vi "validate configuration.vi"(8 "error in":errorcluster, 11 "Tag Bus Web Interface configuration in":refnum<class "Tag Bus Web Interface configuration.lvclass">) -> (0 "error out":errorcluster, 3 "Tag Bus Web Interface configuration out":refnum<class "Tag Bus Web Interface configuration.lvclass">)   [LabVIEW 2013, in "Tag Bus Web Interface configuration.lvclass"]
doc: "This function performs validation of the configuration. This function should be safe to call at any point and should not rely on anything in the runtime environment."
uses:
  Tag Bus Web Interface configuration.lvclass
  <vilib>/NI/Tag Bus Module Framework/module configuration/TBM module configuration.lvclass
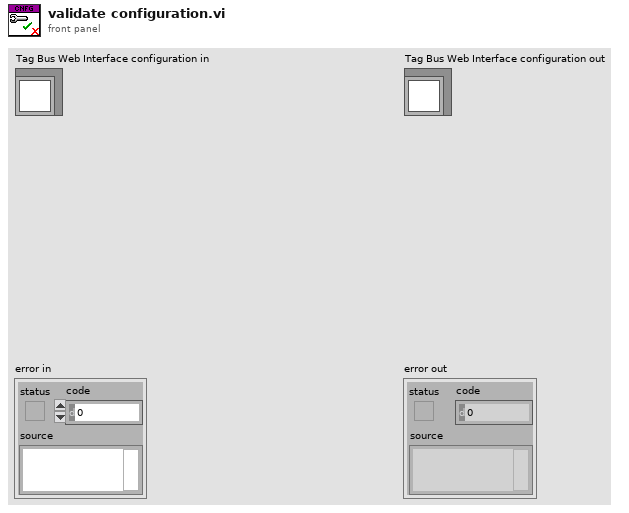
[diagram p1: front panel]
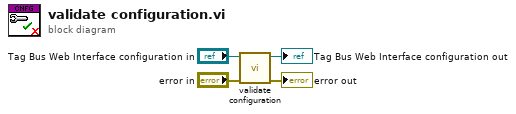
[diagram p0: block diagram]
diagram:
  n1 = call-parent "validate configuration.vi"("error in"="error in", "configuration in"="Tag Bus Web Interface configuration in") -> ("error out"=→"error out":errorcluster, "configuration out"=→"Tag Bus Web Interface configuration out":refnum<class "Tag Bus Web Interface configuration.lvclass">)  [unwired: 8 in]
